vi "GetSet Singleton.vi"(6 "Action":T1, 8 "error in (no error)":errorcluster, 11 "RT Variables in":refnum<class "RT Variables.lvclass">) -> (0 "error out":errorcluster, 3 "RT Variables out":refnum<class "RT Variables.lvclass">)   [LabVIEW 2019, in "LSL.lvlib" / "RT Variables.lvclass"]
uses:
  RT Variables.lvclass
  Singleton Action.ctl
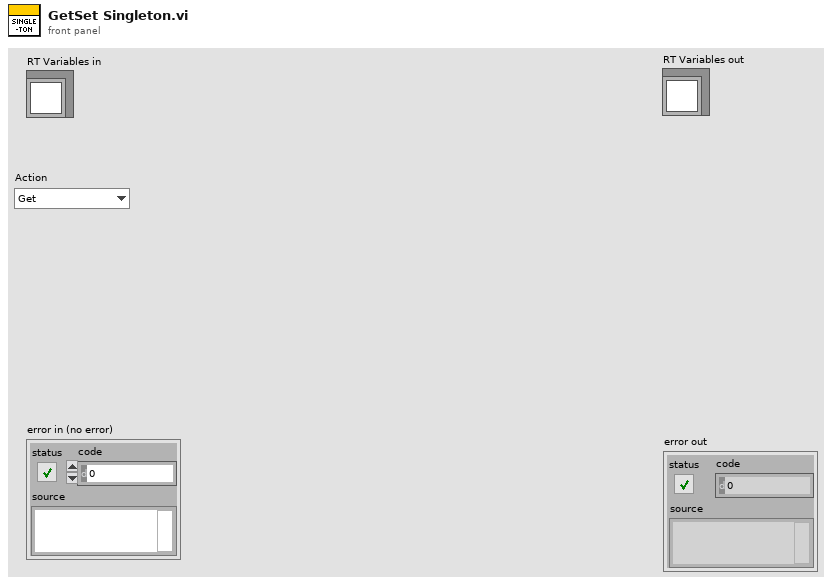
[diagram p1: front panel]
types:
  T1 = typedef "LSL.lvlib/RT Variables.lvclass/Singleton Action.ctl" = enum16{"Get", "Set"}
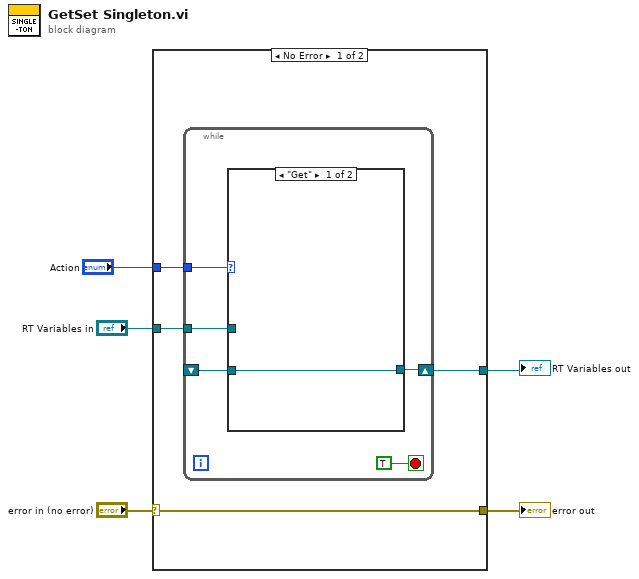
[diagram p0: block diagram]
diagram:
  n1 = case shown="No Error" "error in (no error)" {
    selector: "error in (no error)" -> [w9 w17]
    tunnel: [w9 w17] -> w4
    tunnel: [w6 w18] -> w3
    tunnel: "RT Variables in" -> [w7 w18]
    tunnel: "Action" -> [w8 _]
    frame No Error {
      n2 = while {
        tunnel: w8 -> [w13]
        tunnel: w7 -> [w11]
        shift-right: [w12] -> w6
        shift-left: _ -> [w10]
        stop <- TRUE stop-if-true
        n3 = case shown="\"Get\"" w13 {
          tunnel: [w15 w16] -> w12
          tunnel: w11 -> [_ w16]
          tunnel: w10 -> [w15 _]
          frame "Get" {
          }
          frame "Set" {
          }
        }
      }
    }
    frame Error {
    }
  }
  "error out" <- w4
  "RT Variables out" <- w3
